vi "Build Package.vi"(0 "Destination Path":path, 1 "Package Path":path, 2 "Build Package?":bool, 7 "Package Spec":string[](array[string]), 11 "error in (no error)":errorcluster) -> (4 "Package Directory":path, 6 "Error Message":string, 15 "error out":errorcluster)   [LabVIEW 2021, in "Packager Helpers.lvlib"]
uses:
  Packager Helpers.lvlib
  Path Functions/Path Functions.lvlib
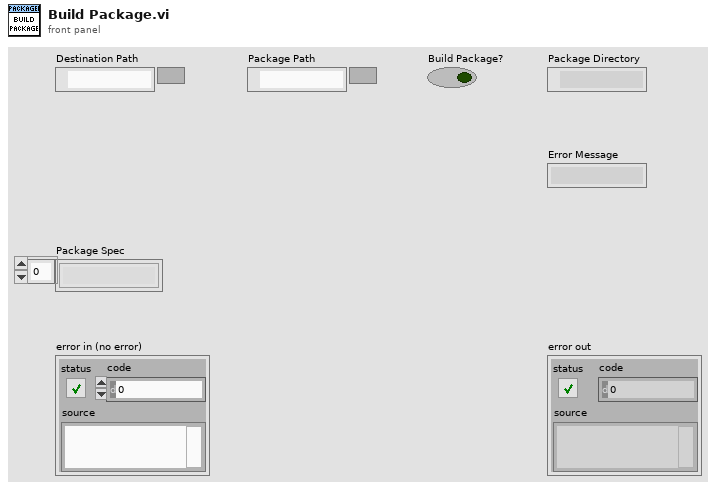
[diagram p1: front panel]
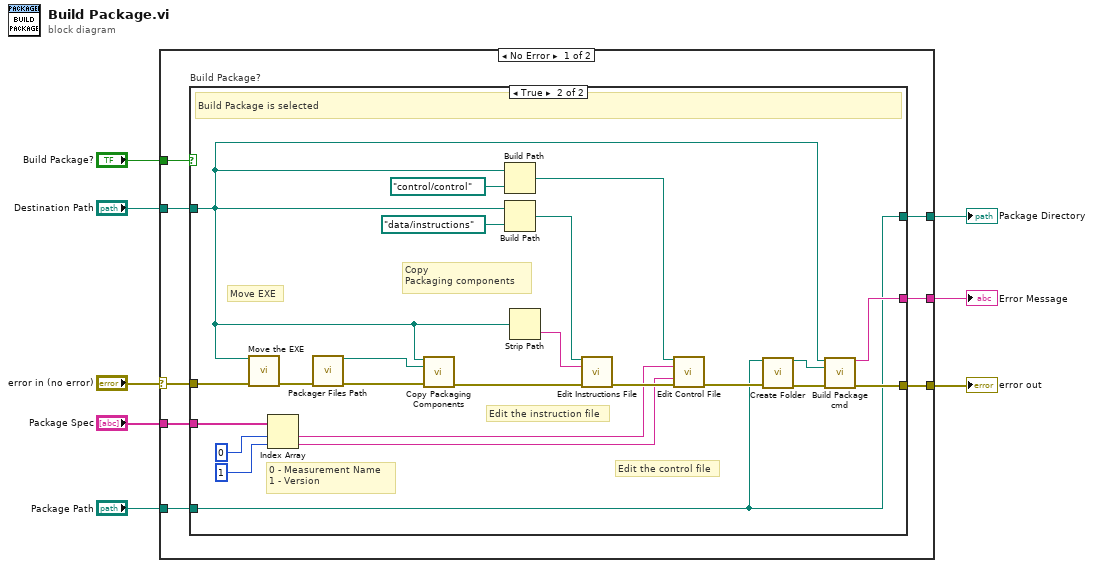
[diagram p0: block diagram]
diagram:
  n1 = case shown="No Error" "error in (no error)" {
    selector: "error in (no error)" -> [w12 w42]
    tunnel: [w16 w42] -> w8
    tunnel: [w15 w41] -> w7
    tunnel: "Destination Path" -> [w14 _]
    tunnel: "Package Spec" -> [w13 _]
    tunnel: "Build Package?" -> [w9 _]
    tunnel: [w11 _] -> w2
    tunnel: "Package Path" -> [w10 w41]
    frame No Error {
      n2 = case "Build Package?" shown="True" w9 {
        tunnel: w12 -> [w17 w27]
        tunnel: w13 -> [_ w32]
        tunnel: w14 -> [_ w19]
        tunnel: [_ w18] -> w15
        tunnel: [w17 w28] -> w16
        tunnel: [_ w29] -> w11
        tunnel: w10 -> [_ w18]
        frame False {
        }
        frame True {
          # "Copy \nPackaging components"
          # "Move EXE"
          # "Edit the control file"
          # "Edit the instruction file"
          # "0 - Measurement Name\n1 - Version"
          # "Build Package is selected"
          n3 = call "Move the EXE.vi"("Primary destination path"=w19, "error in (no error)"=w27) -> ("error out"=w24:errorcluster)  [unwired: 13 in]
          n4 = Index Array(array=w32, index #1=0 ("index"), index #2=1 ("index")) -> (element #1=w22:string, element #2=w23:string)
          n5 = call "Packager Files Path.vi"("error in (no error)"=w24) -> ("Template Path"=w26:path, "error out"=w25:errorcluster)  [unwired: 12 in, 1 out]
          n6 = call "Copy Packaging Components.vi"("Primary destination path"=w19, "Template Path"=w26, "error in (no error)"=w25) -> ("error out"=w33:errorcluster)  [unwired: 11 in, 1 out]
          n7 = Build Path(base path=w19, name or relative path=path "control/control") -> (appended path=w30:path)
          n8 = Build Path(base path=w19, name or relative path=path "data/instructions") -> (appended path=w36:path)
          n9 = Strip Path(path=w19) -> (name=w35:string)  [unwired: 1 out]
          n10 = call "Edit Instructions File.vi"("Instruction File Path"=w36, "Measurement Name"=w35, "error in (no error)"=w33) -> ("error out"=w37:errorcluster)  [unwired: 12 in]
          n11 = call "Edit Control File.vi"("Control File Path"=w30, "Measurement Name"=w22, "Version"=w23, "error in (no error)"=w37) -> ("error out"=w31:errorcluster)  [unwired: 11 in]
          n12 = call "Create Folder.vi"("Directory Path"=w18, "error in (no error)"=w31) -> ("Dup Directory Path"=w21:path, "error out"=w20:errorcluster)  [unwired: 12 in]
          n13 = call "Build Package cmd.vi"("Source Path"=w19, "Destination Dir"=w21, "error in (no error)"=w20) -> ("Error Message"=w29:string, "error out"=w28:errorcluster)  [unwired: 11 in]
        }
      }
    }
    frame Error {
    }
  }
  "error out" <- w8
  "Package Directory" <- w7
  "Error Message" <- w2
